vi "Picture Font.vi"(8 "Default BG":u32(colorbox)=2302755, 9 "Default FG":u32(colorbox)=16448250, 10 "Text Attributes":T1, 11 "Terminal Options":T3={"Implied CR with LF"=TRUE, "Local Echo"=FALSE, "Tab Width"=8, "Color Scheme"={"Black"=2302755, "Red"=16711695, "Green"=9232651, "Yellow"=16759040, "Blue"=36344, "Magenta"=7160742, "Cyan"=55531, "White"=15132390, "Bright Black"=4473924, "Bright Red"=16721728, "Bright Green"=11264347, "Bright Yellow"=16765506, "Bright Blue"=37631, "Bright Magenta"=10117099, "Bright Cyan"=6815728, "Bright White"=16777215}, "Default FG"=37, "Default BG"=90, "History Length"=5000, "Font Face"="Fixedsys", "Font Size"=14, "Rows"=24, "Cols"=80} {"Default BG" items=["Black"=30, "Red"=31, "Green"=32, "Yellow"=33, "Blue"=34, "Magenta"=35, "Cyan"=36, "White"=37, "Gray"=90, "Bright Red"=91, "Bright Green"=92, "Bright Yellow"=93, "Bright Blue"=94, "Bright Magenta"=95, "Bright Cyan"=96, "Bright White"=97]; "Default FG" items=["Black"=30, "Red"=31, "Green"=32, "Yellow"=33, "Blue"=34, "Magenta"=35, "Cyan"=36, "White"=37, "Gray"=90, "Bright Red"=91, "Bright Green"=92, "Bright Yellow"=93, "Bright Blue"=94, "Bright Magenta"=95, "Bright Cyan"=96, "Bright White"=97]}) -> (2 "BG":u32(colorbox), 3 "FG":u32(colorbox), 5 "Picture Font":T2)   [LabVIEW 2020, in "Terminal.lvlib" / "Terminal.lvclass"]
uses:
  Terminal.lvclass
  Terminal Options.ctl
  Color Scheme.ctl
  Color.ctl
  Text Attributes.ctl
  Terminal.lvlib
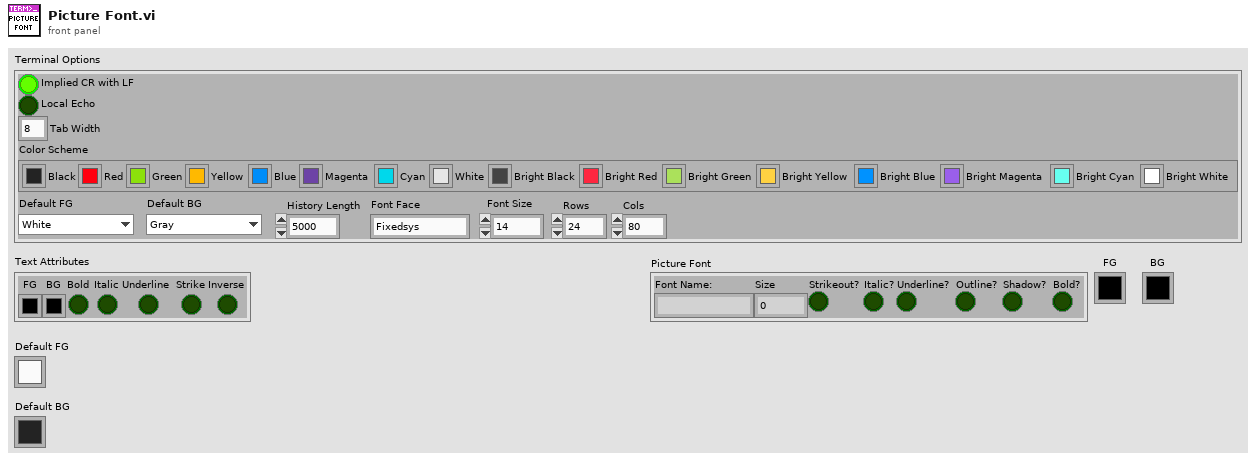
[diagram p1: front panel]
types:
  T1 = typedef "Terminal.lvlib/Text Attributes.ctl" = cluster{"FG":u32, "BG":u32, "Bold":bool, "Italic":bool, "Underline":bool, "Strike":bool, "Inverse":bool}
  T2 = cluster{"Font Name:":string, "Size":i16, "Strikeout?":bool, "Italic?":bool, "Underline?":bool, "Outline?":bool, "Shadow?":bool, "Bold?":bool}
  T3 = typedef "Terminal.lvlib/Terminal Options.ctl" = cluster{"Implied CR with LF":bool, "Local Echo":bool, "Tab Width":i32, "Color Scheme":T4, "Default FG":T5, "Default BG":T5, "History Length":i32, "Font Face":string, "Font Size":i16, "Rows":i32, "Cols":i32}
  T4 = typedef "Terminal.lvlib/Color Scheme.ctl" = cluster{"Black":u32, "Red":u32, "Green":u32, "Yellow":u32, "Blue":u32, "Magenta":u32, "Cyan":u32, "White":u32, "Bright Black":u32, "Bright Red":u32, "Bright Green":u32, "Bright Yellow":u32, "Bright Blue":u32, "Bright Magenta":u32, "Bright Cyan":u32, "Bright White":u32}
  T5 = typedef "Terminal.lvlib/Color.ctl" = i8
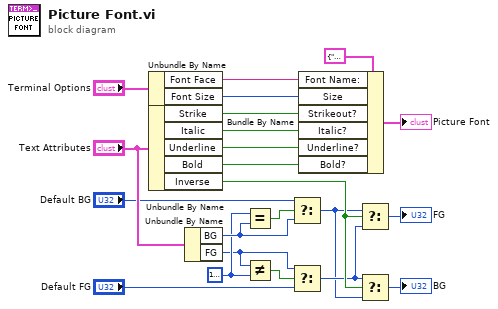
[diagram p0: block diagram]
diagram:
  w4 = u32 16777216
  n1 = Unbundle By Name("Terminal Options") -> ("Font Face"=w16:string, "Font Size"=w17:i16)
  n2 = Unbundle By Name("Text Attributes") -> ("Strike"=w21:bool, "Italic"=w20:bool, "Underline"=w19:bool, "Bold"=w18:bool, "Inverse"=w14:bool)
  n3 = Unbundle By Name("Text Attributes") -> ("BG"=w5:u32, "FG"=w2:u32)
  n4 = Equal?(x=w4, y=w5) -> (x = y?=w3:bool)
  n5 = Not Equal?(x=w2, y=w4) -> (x != y?=w9:bool)
  n6 = Select(t="Default BG", s=w3, f=w5) -> (s? t:f=w1:u32)
  n7 = Select(t=w2, s=w9, f="Default FG") -> (s? t:f=w10:u32)
  n8 = Bundle By Name(cluster=T2 {"Font Name:"="", "Size"=12, "Strikeout?"=FALSE, "Italic?"=FALSE, "Underline?"=FALSE, "Outline?"=FALSE, "Shadow?"=FALSE, "Bold?"=FALSE} ("[user-specified font]"), "Font Name:"=w16, "Size"=w17, "Strikeout?"=w21, "Italic?"=w20, "Underline?"=w19, "Bold?"=w18) -> (→"Picture Font":T2)
  n9 = Select(t=w1, s=w14, f=w10) -> (s? t:f=→"FG":u32)
  n10 = Select(t=w10, s=w14, f=w1) -> (s? t:f=→"BG":u32)
